vi "Test Animation.vi"() -> (3 "Text Output":string)   [LabVIEW 2015]
panel:
  in  "Text Input":string="To login Please Enter your user name & password "
  in  "Reset Timer":bool
  in  "Numeric":i32
  in  "length (rest)":i32
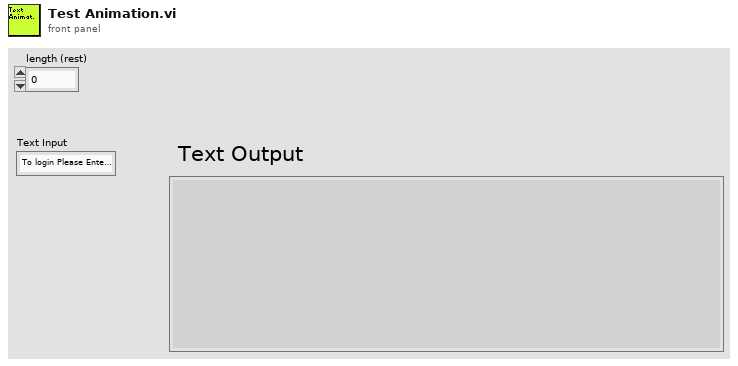
[diagram p1: front panel]
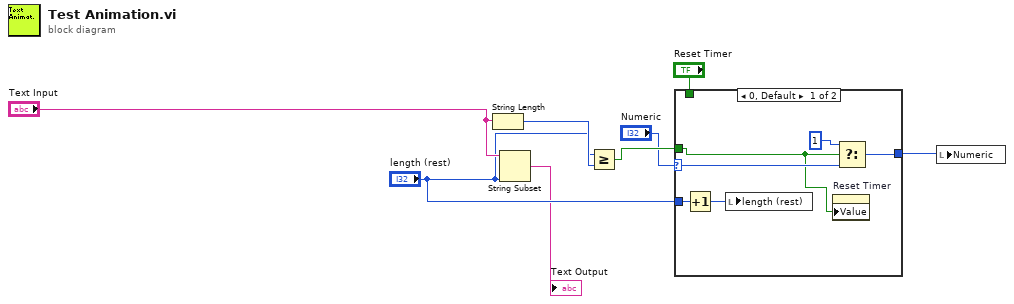
[diagram p0: block diagram]
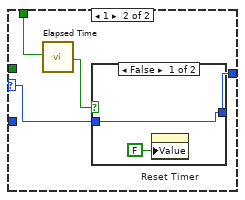
[diagram p2: hidden frame]
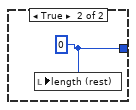
[diagram p3: hidden frame]
diagram:
  n1 = String Length(string="Text Input") -> (length=w7:i32)
  n2 = String Subset(string="Text Input", length (rest)="length (rest)") -> (substring=→"Text Output":string)  [unwired: 1 in]
  n3 = Greater Or Equal?(x="length (rest)", y=w7) -> (x >= y?=w4:bool)
  n4 = case shown="0, Default" "Numeric" {
    selector: "Numeric" -> [w11 w16]
    tunnel: "length (rest)" -> [w14 _]
    tunnel: w4 -> [w9 _]
    tunnel: [w12 w17] -> w2
    tunnel: "Reset Timer" -> [_ w15]
    frame 0, Default {
      n5 = Increment(x=w14) -> (x+1=w13:i32)
      n6 = local write "length (rest)"(w13) -> ()
      n7 = property on="Reset Timer" class="Bool (strict)"("Value"=w9) -> ()  [unwired: 2 in, 2 out]
      n8 = Select(t=1, s=w9, f=w11) -> (s? t:f=w12:i32)
    }
    frame 1 {
      n9 = call "Elapsed Time"("Reset"=w15) -> ("Time has Elapsed"=w18:bool)  [unwired: 11 in, 7 out]
      n10 = case shown="False" w18 {
        tunnel: [w20 w21] -> w17
        tunnel: w16 -> [w20 _]
        frame False {
          n11 = property on="Reset Timer" class="Bool (strict)"("Value"=FALSE ("Reset Timer")) -> ()  [unwired: 2 in, 2 out]
        }
        frame True {
          w21 = 0 ("Numeric")
          n12 = local write "length (rest)"(w21) -> ()
        }
      }
    }
  }
  n13 = local write "Numeric"(w2) -> ()
